vi "Cluster is one element or unnamed elements.vi"(9 "Cluster Elements Array":T1[](array[typedef]), 11 "Cluster Terminal":refnum<vi>) -> (1 "Some Unnamed?":bool, 2 "All Unnamed?":bool, 3 "One Element?":bool)   [LabVIEW 2023]
doc: "Reports if cluster data has one element, which is unnamed, has \"all\" unnamed elements, which for our purposes means all parent items are unnamed (since child items can't be named without a named parent), or has some items unnamed, meaning at least some items can be programtically manipulated by name.\n\nThis VI works on a reference OR an array of cluster element descriptions."
uses:
  Cluster Element Description.ctl
  <vilib>/Utility/Data Type/NI_Data Type.lvlib
  <userlib>/_OpenG.lib/array/array.llb/openg_array.lvlib
panel:
  # "Uses one of these inputs"
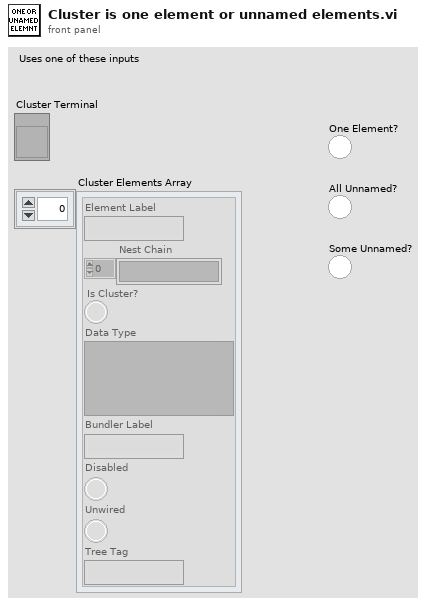
[diagram p1: front panel]
types:
  T1 = typedef "Cluster Element Description.ctl" = cluster{"Element Label":string, "Nest Chain":string[], "Is Cluster?":bool, "Data Type":variant, "Bundler Label":string, "Disabled":bool, "Unwired":bool, "Tree Tag":string}
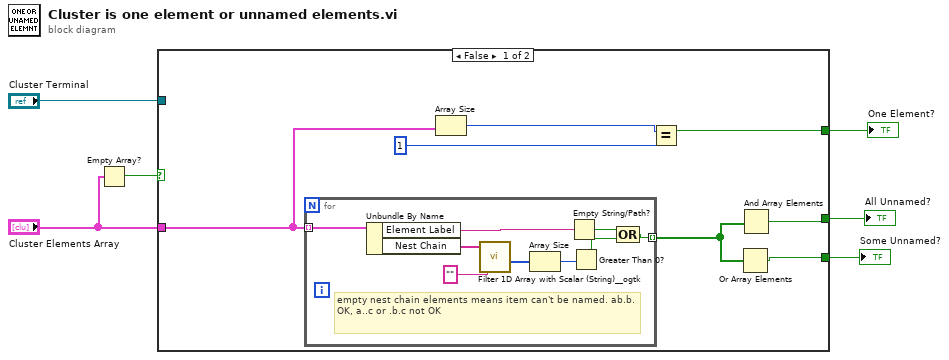
[diagram p0: block diagram]
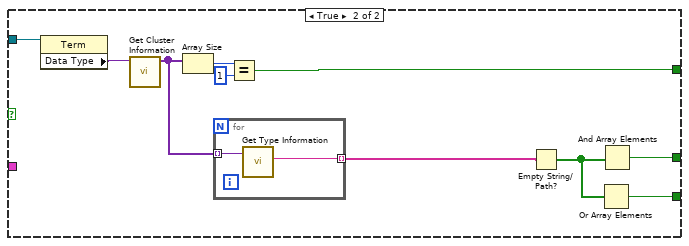
[diagram p2: hidden frame]
diagram:
  n1 = Empty Array?(array="Cluster Elements Array") -> (empty?=w3:bool)
  n2 = case shown="False" w3 {
    tunnel: [w11 w32] -> w6
    tunnel: [w9 w27] -> w5
    tunnel: [w8 w25] -> w4
    tunnel: "Cluster Elements Array" -> [w10 _]
    tunnel: "Cluster Terminal" -> [_ w23]
    frame False {
      n3 = for {
        tunnel: w10 -> [w22] mode=indexing
        tunnel: [w14] -> w7 mode=indexing
        # "empty nest chain elements means item can't be named. ab.b. OK, a..c or .b.c not OK"
        n4 = Unbundle By Name(w22) -> ("Element Label"=w17:string, "Nest Chain"=w21:string[])
        n5 = call <userlib>:"Filter 1D Array with Scalar (String)__ogtk.vi"("items to filter"="" ("String"), "array"=w21) -> ("filtered item indices"=w19:i32[])  [unwired: 4 in, 1 out]
        n6 = Array Size(array=w19) -> (size(s)=w18:i32)
        n7 = Empty String/Path?(string/path=w17) -> (empty?=w16:bool)
        n8 = Greater Than 0?(x=w18) -> (x > 0?=w15:bool)
        n9 = Compound Arithmetic op=OR(w16, w15) -> (w14:bool)
      }
      n10 = Array Size(array=w10) -> (size(s)=w13:i32)
      n11 = Equal?(x=w13, y=1) -> (x = y?=w11:bool)
      n12 = Or Array Elements(Boolean array=w7) -> (logical OR=w8:bool)
      n13 = And Array Elements(Boolean array=w7) -> (logical AND=w9:bool)
    }
    frame True {
      n14 = property class="Term"(reference=w23) -> ("Data Type"=w24:variant)  [unwired: 1 in, 2 out]
      n15 = call <vilib>:"Get Cluster Information.vi"("variant"=w24) -> ("cluster elements"=w29:variant[])  [unwired: 9 in, 1 out]
      n16 = Array Size(array=w29) -> (size(s)=w30:i32)
      n17 = for {
        tunnel: w29 -> [w34] mode=indexing
        tunnel: [w33] -> w28 mode=indexing
        n18 = call <vilib>:"Get Type Information.vi"("variant"=w34) -> ("name"=w33:string)  [unwired: 6 in, 4 out]
      }
      n19 = Equal?(x=w30, y=1) -> (x = y?=w32:bool)
      n20 = Empty String/Path?(string/path=w28) -> (empty?=w26:bool[])
      n21 = Or Array Elements(Boolean array=w26) -> (logical OR=w25:bool)
      n22 = And Array Elements(Boolean array=w26) -> (logical AND=w27:bool)
    }
  }
  "One Element?" <- w6
  "All Unnamed?" <- w5
  "Some Unnamed?" <- w4
